vi "Configure Glitch Trigger Source [GT] Core.vi"(0 "CS++Scope":refnum<class "CS++Scope.lvclass">, 1 "trigger source (\"CHANNEL1\")":string(combo)="CHANNEL1", 2 "trigger level (0.0 V)":dbl[unit] format="%.3f", 3 "glitch width (10 ms)":dbl[unit]=1e-05 format="%^.2e", 4 "glitch polarity (Positive)":i32(ring)=1 items=["Positive"=1, "Negative"=2, "Either"=3], 5 "error in (no error)":errorcluster, 6 "glitch condition (Less Than)":i32(ring)=1 items=["Less Than"=1, "Greater Than"=2]) -> (14 "CS++Scope out":refnum<class "CS++Scope.lvclass">, 19 "error out":errorcluster)   [LabVIEW 2014, in "CS++Scope.lvlib" / "CS++Scope.lvclass"]
doc: "This VI configures the glitch trigger. A glitch trigger occurs when the trigger signal has a pulse with a width that is less than or greater than the glitch width. You specifiy which comparison criterion to use with the glitchCondition parameter. You specifiy the glitch width in the glitchWidth parameter. You specifiy the polarity of the pulse with the glitchPolarity parameter. The trigger does not actually occur until the edge of a pulse that corresponds to the glitchWidth and glitchPolarity crosses the threshold the end-user specifies in the triggerLevel parameter.\n\nNote:\nThis VI affects instrument behavior only if the trigger type is IVISCOPE_VAL_GLITCH_TRIGGER. Call the IviScope Configure Trigger and IviScope Configure Trigger Coupling VIs to set the trigger type and trigger coupling before calling this VI."
uses:
  CS++Scope.lvclass
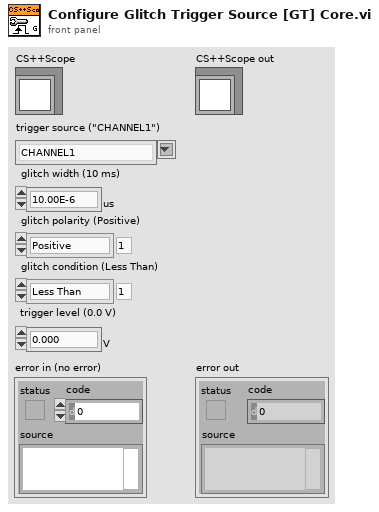
[diagram p1: front panel]
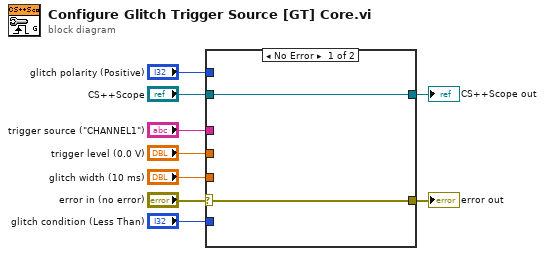
[diagram p0: block diagram]
diagram:
  n1 = case shown="No Error" "error in (no error)" {
    selector: "error in (no error)" -> [w10 w13]
    tunnel: [w10 w13] -> w8
    tunnel: [w11 w12] -> w2
    tunnel: "CS++Scope" -> [w11 w12]
    tunnel: "trigger source (\"CHANNEL1\")" -> [_ _]
    tunnel: "trigger level (0.0 V)" -> [_ _]
    tunnel: "glitch width (10 ms)" -> [_ _]
    tunnel: "glitch polarity (Positive)" -> [_ _]
    tunnel: "glitch condition (Less Than)" -> [_ _]
    frame No Error {
    }
    frame Error {
    }
  }
  "error out" <- w8
  "CS++Scope out" <- w2
